vi "Tetra_AntSel.vi"(0 "COMPORT":refnum<visa-resource-name>="COM4", 3 "REVC(T)":bool=TRUE, 5 "error in (no error)":errorcluster, 6 "RO(t)":bool, 7 "RX/TX":i32(ring)=1 items=["RX", "TX"], 8 "VERIFY(t)":bool, 9 "ANT(num)":i32=1 min=0 max=12 step=1, 11 "Open Ser(t)":bool, 12 "milliseconds to wait":u32, 13 "Close Ser(t)":bool) -> (10 "ant(num)":i32=1, 14 "comport":refnum<visa-resource-name>="COM4", 19 "error out":errorcluster)   [LabVIEW 2018]
panel:
  out "output":string
  out "Ant(name)":string
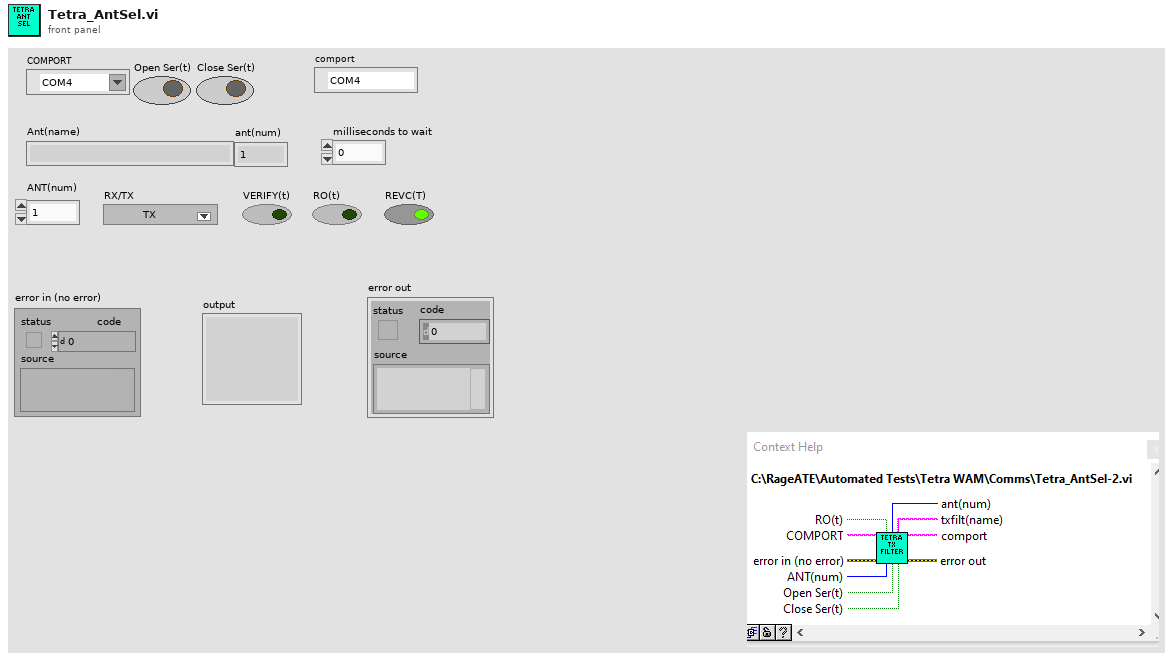
[diagram p1: front panel]
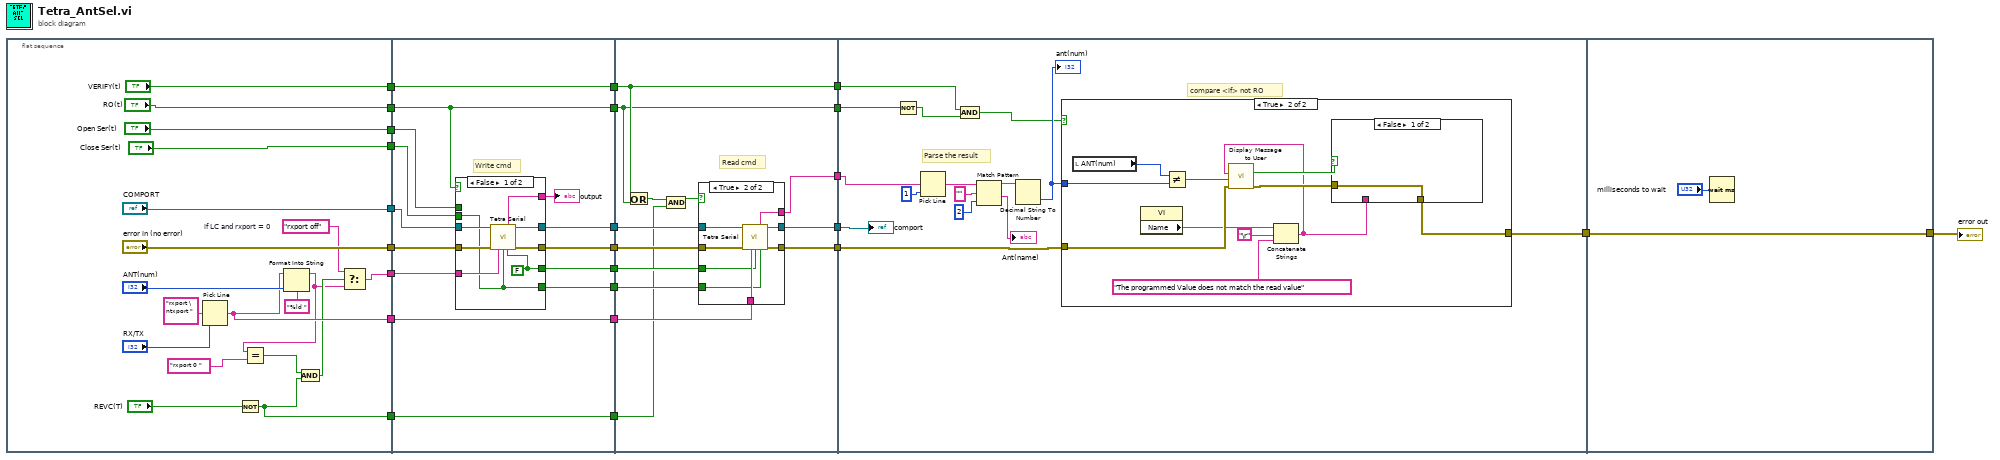
[diagram p0: block diagram]
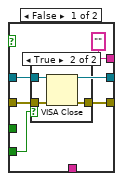
[diagram p3: hidden frame]
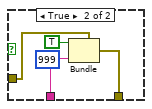
[diagram p6: hidden frame]
diagram:
  n1 = flat-sequence {
    tunnel: ["error in (no error)"] -> w24
    tunnel: ["COMPORT"] -> w23
    tunnel: [w30] -> w22
    tunnel: ["Open Ser(t)"] -> w21
    tunnel: [w33] -> w20
    tunnel: ["Close Ser(t)"] -> w19
    tunnel: ["RO(t)"] -> w13
    tunnel: ["VERIFY(t)"] -> w11
    tunnel: [w25] -> w2
    tunnel: w24 -> [w56]
    tunnel: w23 -> [w55]
    tunnel: w22 -> [w54]
    tunnel: w21 -> [w53]
    tunnel: w20 -> [w57]
    tunnel: w19 -> [w50]
    tunnel: [w57] -> w18
    tunnel: [w52] -> w17
    tunnel: [w51] -> w16
    tunnel: w13 -> [w46]
    tunnel: [w49] -> w12
    tunnel: w11 -> [w49]
    tunnel: [w48] -> w9
    tunnel: [w47] -> w8
    tunnel: [w46] -> w6
    tunnel: w2 -> [w44]
    tunnel: [w44] -> w1
    tunnel: w18 -> [w80]
    tunnel: w17 -> [w81]
    tunnel: w16 -> [w82]
    tunnel: [w79] -> w15
    tunnel: [w78] -> w14
    tunnel: w12 -> [w75]
    tunnel: [w75] -> w10
    tunnel: w9 -> [w77]
    tunnel: w8 -> [w76]
    tunnel: [w74] -> w7
    tunnel: w6 -> [w74]
    tunnel: [w73] -> w3
    tunnel: w1 -> [w70]
    tunnel: w15 -> [w106]
    tunnel: w14 -> [w105]
    tunnel: w10 -> [w104]
    tunnel: w7 -> [w102]
    tunnel: [w100] -> w5
    tunnel: w3 -> [w107]
    tunnel: w5 -> [w134]
    tunnel: [w134] -> w4
    frame #0 {
      w27 = "rxport off"  # if LC and rxport = 0
      n2 = Pick Line(multi-line string="rxport \ntxport ", line index="RX/TX") -> (output string=w33:string)  [unwired: 1 in]
      n3 = Not(x="REVC(T)") -> (.not. x?=w25:bool)
      n4 = Format Into String(format string="%ld ", initial string=w33, "ANT(num)") -> (resulting string=w26:string)  [unwired: 1 in, 1 out]
      n5 = Equal?(x=w26, y="rxport 0 ") -> (x = y?=w31:bool)
      n6 = And(x=w31, y=w25) -> (x .and. y?=w28:bool)
      n7 = Select(t=w27, s=w28, f=w26) -> (s? t:f=w30:string)
    }
    frame #1 {
      # "Write cmd"
      n8 = case shown="False" w46 {
        tunnel: w56 -> [w65 w69]
        tunnel: w55 -> [w64 w68]
        tunnel: w54 -> [w63 _]
        tunnel: w53 -> [_ w66]
        tunnel: [w62 w69] -> w52
        tunnel: [w61 w68] -> w51
        tunnel: w50 -> [w59 w67]
        tunnel: [w59 w67] -> w47
        tunnel: [w60 w66] -> w48
        tunnel: [w58 _] -> w45
        frame False {
          w60 = FALSE
          n9 = call "Tetra Serial.vi"("COMPORT"=w64, "error in (no error)"=w65, "Command"=w63, "Open Ser(t)"=w59, "Close Ser(t)"=w60) -> ("output"=w58:string, "comport"=w61:refnum<visa-resource-name>, "error out"=w62:errorcluster)  [unwired: 6 in, 2 out]
        }
        frame True {
        }
      }
      "output" <- w45
    }
    frame #2 {
      # "Read cmd"
      n10 = Or(x=w75, y=w74) -> (x .or. y?=w71:bool)
      n11 = And(x=w71, y=w70) -> (x .and. y?=w72:bool)
      n12 = case shown="True" w72 {
        tunnel: w82 -> [w83 w99]
        tunnel: w81 -> [w87 w98]
        tunnel: w80 -> [_ w97]
        tunnel: ["" ("output") w96] -> w73
        tunnel: [w83 w95] -> w79
        tunnel: [w86 w94] -> w78
        tunnel: w77 -> [_ w93]
        tunnel: w76 -> [w84 w92]
        frame False {
          n13 = case shown="True" w84 {
            tunnel: w87 -> [w88 w91]
            tunnel: [w88 w90] -> w86
            tunnel: w83 -> [_ w89]
            frame False {
            }
            frame True {
              n14 = VISA Close(VISA resource name=w89, error in (no error)=w91) -> (error out=w90:errorcluster)
            }
          }
        }
        frame True {
          n15 = call "Tetra Serial.vi"("COMPORT"=w99, "error in (no error)"=w98, "Command"=w97, "Open Ser(t)"=w93, "Close Ser(t)"=w92) -> ("output"=w96:string, "comport"=w95:refnum<visa-resource-name>, "error out"=w94:errorcluster)  [unwired: 6 in, 2 out]
        }
      }
    }
    frame #3 {
      # "Parse the result"
      # "compare <if> not RO"
      n16 = Not(x=w102) -> (.not. x?=w103:bool)
      n17 = Pick Line(multi-line string=w107, line index=1) -> (output string=w112:string)  [unwired: 1 in]
      n18 = And(x=w104, y=w103) -> (x .and. y?=w101:bool)
      n19 = Match Pattern(string=w112, regular expression="", offset (0)=2) -> (before substring=w114:string, after substring=→"Ant(name)":string)  [unwired: 2 out]
      n20 = Decimal String To Number(string=w114) -> (number=w111:i32)  [unwired: 2 in, 1 out]
      "ant(num)" <- w111
      n21 = case shown="True" w101 {
        tunnel: w111 -> [_ w125]
        tunnel: w105 -> [w115 w124]
        tunnel: [w115 w122] -> w100
        frame False {
        }
        frame True {
          n22 = local read "ANT(num)"() -> (w126:i32)
          n23 = property class="VI"() -> ("Name"=w121:string)  [unwired: 2 in, 2 out]
          n24 = Not Equal?(x=w126, y=w125) -> (x != y?=w120:bool)
          n25 = Concatenate Strings(w121, "\r", "The programmed Value does not match the read value" ("Message")) -> (w118:string)
          n26 = call "Display Message to User"("error in (no error)"=w124, "Enable"=w120, "Message"=w118) -> ("error out"=w123:errorcluster, "OK"=w119:bool)  [unwired: 7 in]
          n27 = case shown="False" w119 {
            tunnel: w123 -> [w127 w131]
            tunnel: [w127 w132] -> w122
            tunnel: w118 -> [_ w130]
            frame False {
            }
            frame True {
              n28 = Bundle(cluster=w131, "status"=TRUE, "code"=999, "source"=w130) -> (w132:errorcluster)
            }
          }
        }
      }
      "comport" <- w106
    }
    frame #4 {
      n29 = Wait (ms)(milliseconds to wait="milliseconds to wait") -> ()  [unwired: 1 out]
    }
  }
  "error out" <- w4
